vi "read_data (SubVI).vi"(11 "data tasks":T2) -> (0 "sample rate":dbl, 1 "Rescaled data":i16[][](array[numeric]), 2 "Output data":dbl[][](array[numeric]), 3 "output data tasks":T1)   [LabVIEW 2018]
uses:
  <vilib>/DAQmx/read.llb/DAQmx Read (Analog 2D DBL NChan NSamp).vi
  <vilib>/DAQmx/read.llb/DAQmx Read (Analog 1D Wfm NChan NSamp).vi
  <vilib>/DAQmx/miscellaneous.llb/DAQmx Fill In Error Info.vi
panel:
  out "data":dbl[][](graph)
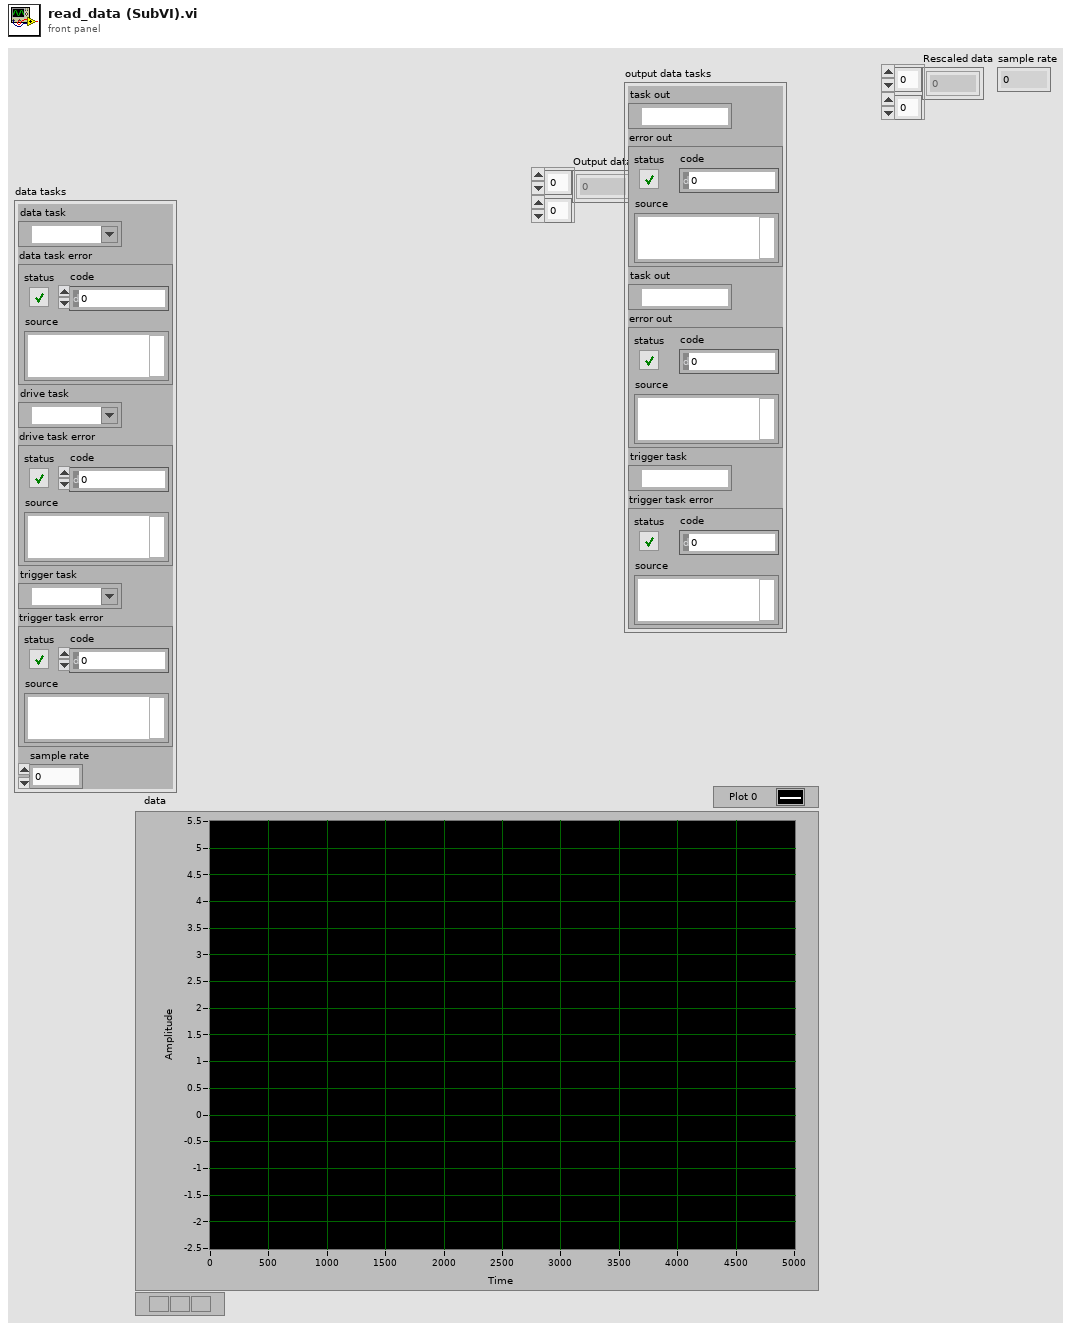
[diagram p1: front panel]
types:
  T1 = cluster{"task out":refnum<k21>, "error out":errorcluster, "task out":refnum<k21>, "error out":errorcluster, "trigger task":refnum<k21>, "trigger task error":errorcluster}
  T2 = cluster{"data task":refnum<k21>, "data task error":errorcluster, "drive task":refnum<k21>, "drive task error":errorcluster, "trigger task":refnum<k21>, "trigger task error":errorcluster, "sample rate":dbl}
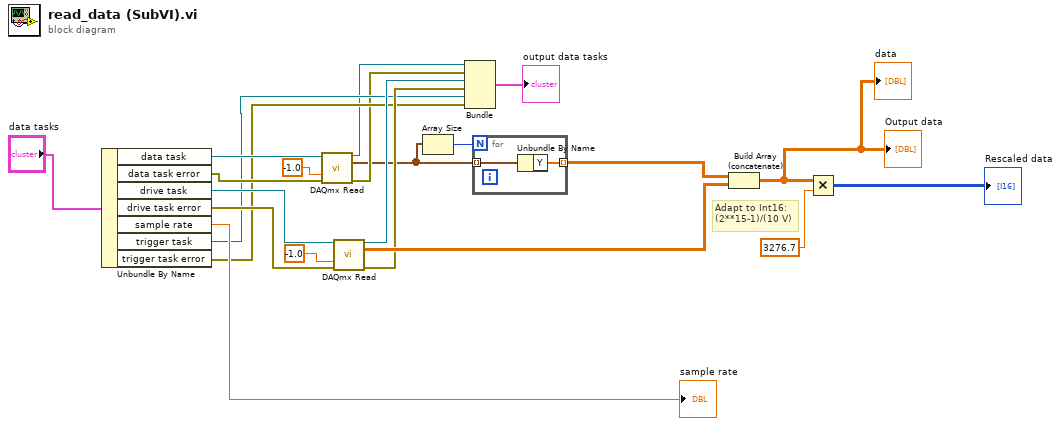
[diagram p0: block diagram]
diagram:
  # "Adapt to Int16: \n(2**15-1)/(10 V)"
  n1 = Unbundle By Name("data tasks") -> ("data task"=w21:refnum<k21>, "data task error"=w20:errorcluster, "drive task"=w18:refnum<k21>, "drive task error"=w17:errorcluster, "sample rate"=→"sample rate":dbl, "trigger task"=w10:refnum<k21>, "trigger task error"=w9:errorcluster)
  n2 = call-poly <vilib>:"DAQmx Read.vi"("task/channels in"=w21, "timeout"=-1.0, "error in"=w20) -> ("task out"=w6:refnum<k21>, "data"=w2:waveform(dbl)[], "error out"=w5:errorcluster)  [unwired: 10 in]
  n3 = call-poly <vilib>:"DAQmx Read.vi"("task/channels in"=w18, "timeout"=-1.0, "error in"=w17) -> ("task out"=w12:refnum<k21>, "data"=w15:dbl[][], "error out"=w11:errorcluster)  [unwired: 10 in]
  n4 = Array Size(array=w2) -> (size(s)=w3:i32)
  n5 = Bundle("task out"=w6, "error out"=w5, "task out"=w12, "error out"=w11, "trigger task"=w10, "trigger task error"=w9) -> (→"output data tasks":T1)  [unwired: 1 in]
  n6 = for {
    N: w3 -> [_]
    tunnel: w2 -> [w24] mode=indexing
    tunnel: [w23] -> w1 mode=indexing
    n7 = Unbundle By Name(w24) -> ("Y"=w23:dbl[])
  }
  n8 = Build Array (concatenate)(w1, w15) -> (w4:dbl[][])
  "Output data" <- w4
  "data" <- w4
  n9 = Multiply(x=w4, y=3276.7) -> (x*y=→"Rescaled data":i16[][])
